vi "WPI_EncoderOpen.vi"(4 "DistancePerCount":dbl=1.0, 5 "External Reset Active High":bool=TRUE, 6 "Decoding Type":T1=enum."4x", 7 "External Reset":T2={"DevStatus"={"status"=FALSE, "code"=0, "source"=""}, "AnalogTriggerMode?"=FALSE, "DigitalMode"={"DIO Channel"=enum."Disabled"}, "AnalogTriggerMode"={"AnalogTriggerIndex"=enum."Trig 0", "OutputType"=enum."InWindow"}}, 8 "error in (no error)":errorcluster, 9 "Invert Direction (False)":bool, 10 "BSource":T2={"DevStatus"={"status"=FALSE, "code"=0, "source"=""}, "AnalogTriggerMode?"=FALSE, "DigitalMode"={"DIO Channel"=enum."Disabled"}, "AnalogTriggerMode"={"AnalogTriggerIndex"=enum."Trig 0", "OutputType"=enum."InWindow"}}, 11 "ASource":T2={"DevStatus"={"status"=FALSE, "code"=0, "source"=""}, "AnalogTriggerMode?"=FALSE, "DigitalMode"={"DIO Channel"=enum."Disabled"}, "AnalogTriggerMode"={"AnalogTriggerIndex"=enum."Trig 0", "OutputType"=enum."InWindow"}}) -> (0 "error out":errorcluster, 3 "EncoderDevRef":T6={"DevStatus"={"status"=FALSE, "code"=0, "source"=""}, "EncoderIndex"=enum."Invalid", "CounterIndex"=enum."Invalid", "DistancePerCount"=1.0, "Decoding Type"=enum."4x"})   [LabVIEW 2017]
doc: "Opens a reference to the encoder you specify. You must open a reference before using any other VIs on this palette.\n\nUse the ToDigitalSource VI to create a digital source that you can wire to the <B>ASource</B> and <B>BSource</B> inputs of this VI. After you open a reference to the encoder, you can use the Start and Stop VIs to start and stop the encoder, respectively.\n\nThis software is licensed. Open the labview\\readme\\WPI Robotics Library Open Source License.txt file for more information."
uses:
  <vilib>/Rock Robotics/SystemInterfaces/Encoder/FPGA_EncoderIdx.ctl
  <vilib>/Rock Robotics/WPI/Encoder/WPI_EncoderDevRef.ctl
  <vilib>/Rock Robotics/WPI/Encoder/WPI_EncoderCacheOp.ctl
  <vilib>/Rock Robotics/WPI/Encoder/WPI_EncoderType.ctl
  <vilib>/Rock Robotics/SystemInterfaces/Counter/FPGA_CounterCtrEdgeDetectionType.ctl
  <vilib>/Rock Robotics/SystemInterfaces/Counter/FPGA_CounterCtrSystemIndex.ctl
  <vilib>/Rock Robotics/SystemInterfaces/Encoder/FPGA_EncoderOpen & Configure.vi
  <instrlib>/Maxon Encoder/HAIOL/Simulator/Maxon Encoder Simulator.lvclass
  <vilib>/robotics/Simulator/Engine/ctl/DeviceID.ctl
  <vilib>/robotics/Simulator/NI_Robotics_Simulator.lvlib
  <vilib>/Rock Robotics/SystemInterfaces/DIO/FPGA_DIOPWMChannel.ctl
  <vilib>/Rock Robotics/SystemInterfaces/AnalogTrigger/FPGA_AnalogTriggerOutType.ctl
  <vilib>/Rock Robotics/SystemInterfaces/CounterEncoderSourceConvertion/FPGA_CounterEncoderSourceConvertionLVSourceType.ctl
  <vilib>/Rock Robotics/SystemInterfaces/DIO/FPGA_DIODigitalSourceChannel.ctl
  <vilib>/Rock Robotics/SystemInterfaces/AnalogTrigger/FPGA_AnalogTriggerIndex.ctl
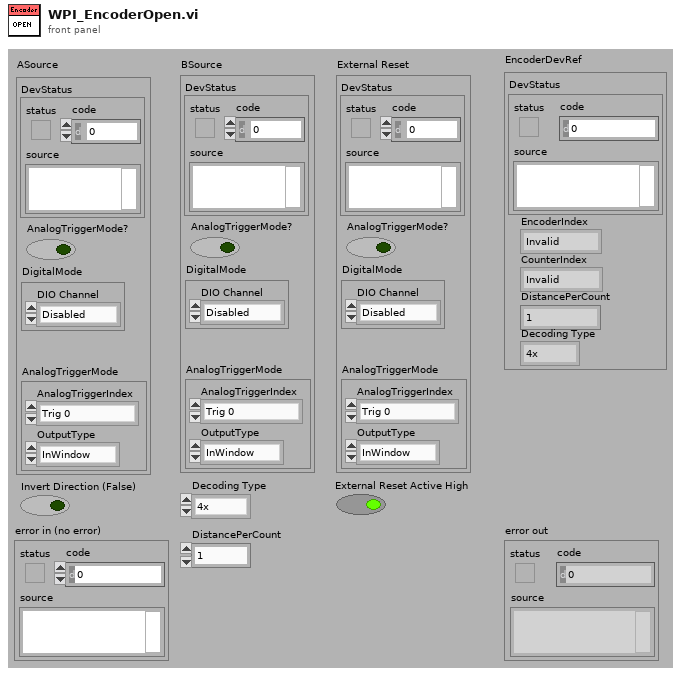
[diagram p1: front panel]
types:
  T1 = typedef "WPI_EncoderType.ctl" = enum16{"1x", "2x", "4x"}
  T2 = typedef "FPGA_CounterEncoderSourceConvertionLVSourceType.ctl" = cluster{"DevStatus":errorcluster, "AnalogTriggerMode?":bool, "DigitalMode":cluster{"DIO Channel":T3}, "AnalogTriggerMode":cluster{"AnalogTriggerIndex":T4, "OutputType":T5}}
  T3 = typedef "FPGA_DIODigitalSourceChannel.ctl" = enum8{"DIO 0", "DIO 1", "DIO 2", "DIO 3", "DIO 4", "DIO 5", "DIO 6", "DIO 7", "DIO 8", "DIO 9", "DIO MXP 0", "DIO MXP 1", "DIO MXP 2", "DIO MXP 3", "DIO MXP 4", "DIO MXP 5", "DIO MXP 6", "DIO MXP 7", "DIO MXP 8", "DIO MXP 9", "DIO MXP 10", "DIO MXP 11", "DIO MXP 12", "DIO MXP 13", "DIO MXP 14", "DIO MXP 15", "Disabled"}
  T4 = typedef "FPGA_AnalogTriggerIndex.ctl" = enum8{"Trig 0", "Trig 1", "Trig 2", "Trig 3", "Trig 4", "Trig 5", "Trig 6", "Trig 7", "Invalid"}
  T5 = typedef "FPGA_AnalogTriggerOutType.ctl" = enum16{"InWindow", "TriggerState", "Rising", "Falling"}
  T6 = typedef "WPI_EncoderDevRef.ctl" = cluster{"DevStatus":errorcluster, "EncoderIndex":T7, "CounterIndex":T8, "DistancePerCount":dbl, "Decoding Type":T1}
  T7 = typedef "FPGA_EncoderIdx.ctl" = enum8{"Enc 0", "Enc 1", "Enc 2", "Enc 3", "Enc 4", "Enc 5", "Enc 6", "Enc 7", "Invalid"}
  T8 = typedef "FPGA_CounterCtrSystemIndex.ctl" = enum8{"Ctr 0", "Ctr 1", "Ctr 2", "Ctr 3", "Ctr 4", "Ctr 5", "Ctr 6", "Ctr 7", "Invalid"}
  T9 = typedef "FPGA_CounterCtrEdgeDetectionType.ctl" = cluster{"Master Mode":enum16{"Edge Detection", "Semi Period Mode", "Pulse Length Mode", "External Direction"}, "UpChannel":enum16{"Rising Edge", "Falling Edge", "Raising & Falling Edge", "Disabled"}, "DownChannel":enum16{"Rising Edge", "Falling Edge", "Raising & Falling Edge", "Disabled"}, "High/Up":bool}
  T10 = enum16{"Rising Edge", "Falling Edge", "Raising & Falling Edge", "Disabled"}
  T11 = typedef "WPI_EncoderCacheOp.ctl" = enum16{"Acquire", "Release"}
  T12 = typedef "FPGA_DIOPWMChannel.ctl" = enum8{"PWM 0", "PWM 1", "PWM 2", "PWM 3", "PWM 4", "PWM 5", "PWM 6", "PWM 7", "PWM 8", "PWM 9", "PWM MXP 0", "PWM MXP 1", "PWM MXP 2", "PWM MXP 3", "PWM MXP 4", "PWM MXP 5", "PWM MXP 6", "PWM MXP 7", "PWM MXP 8", "PWM MXP 9", "Invalid"}
  T13 = typedef "NI_Robotics_Simulator.lvlib/DeviceID.ctl" = cluster{"robot ID":string, "sensor/actuator ID":string}
  T14 = typedef "WPI_CounterDevRef.ctl" = cluster{"DevStatus":errorcluster, "CntIndex":T8}
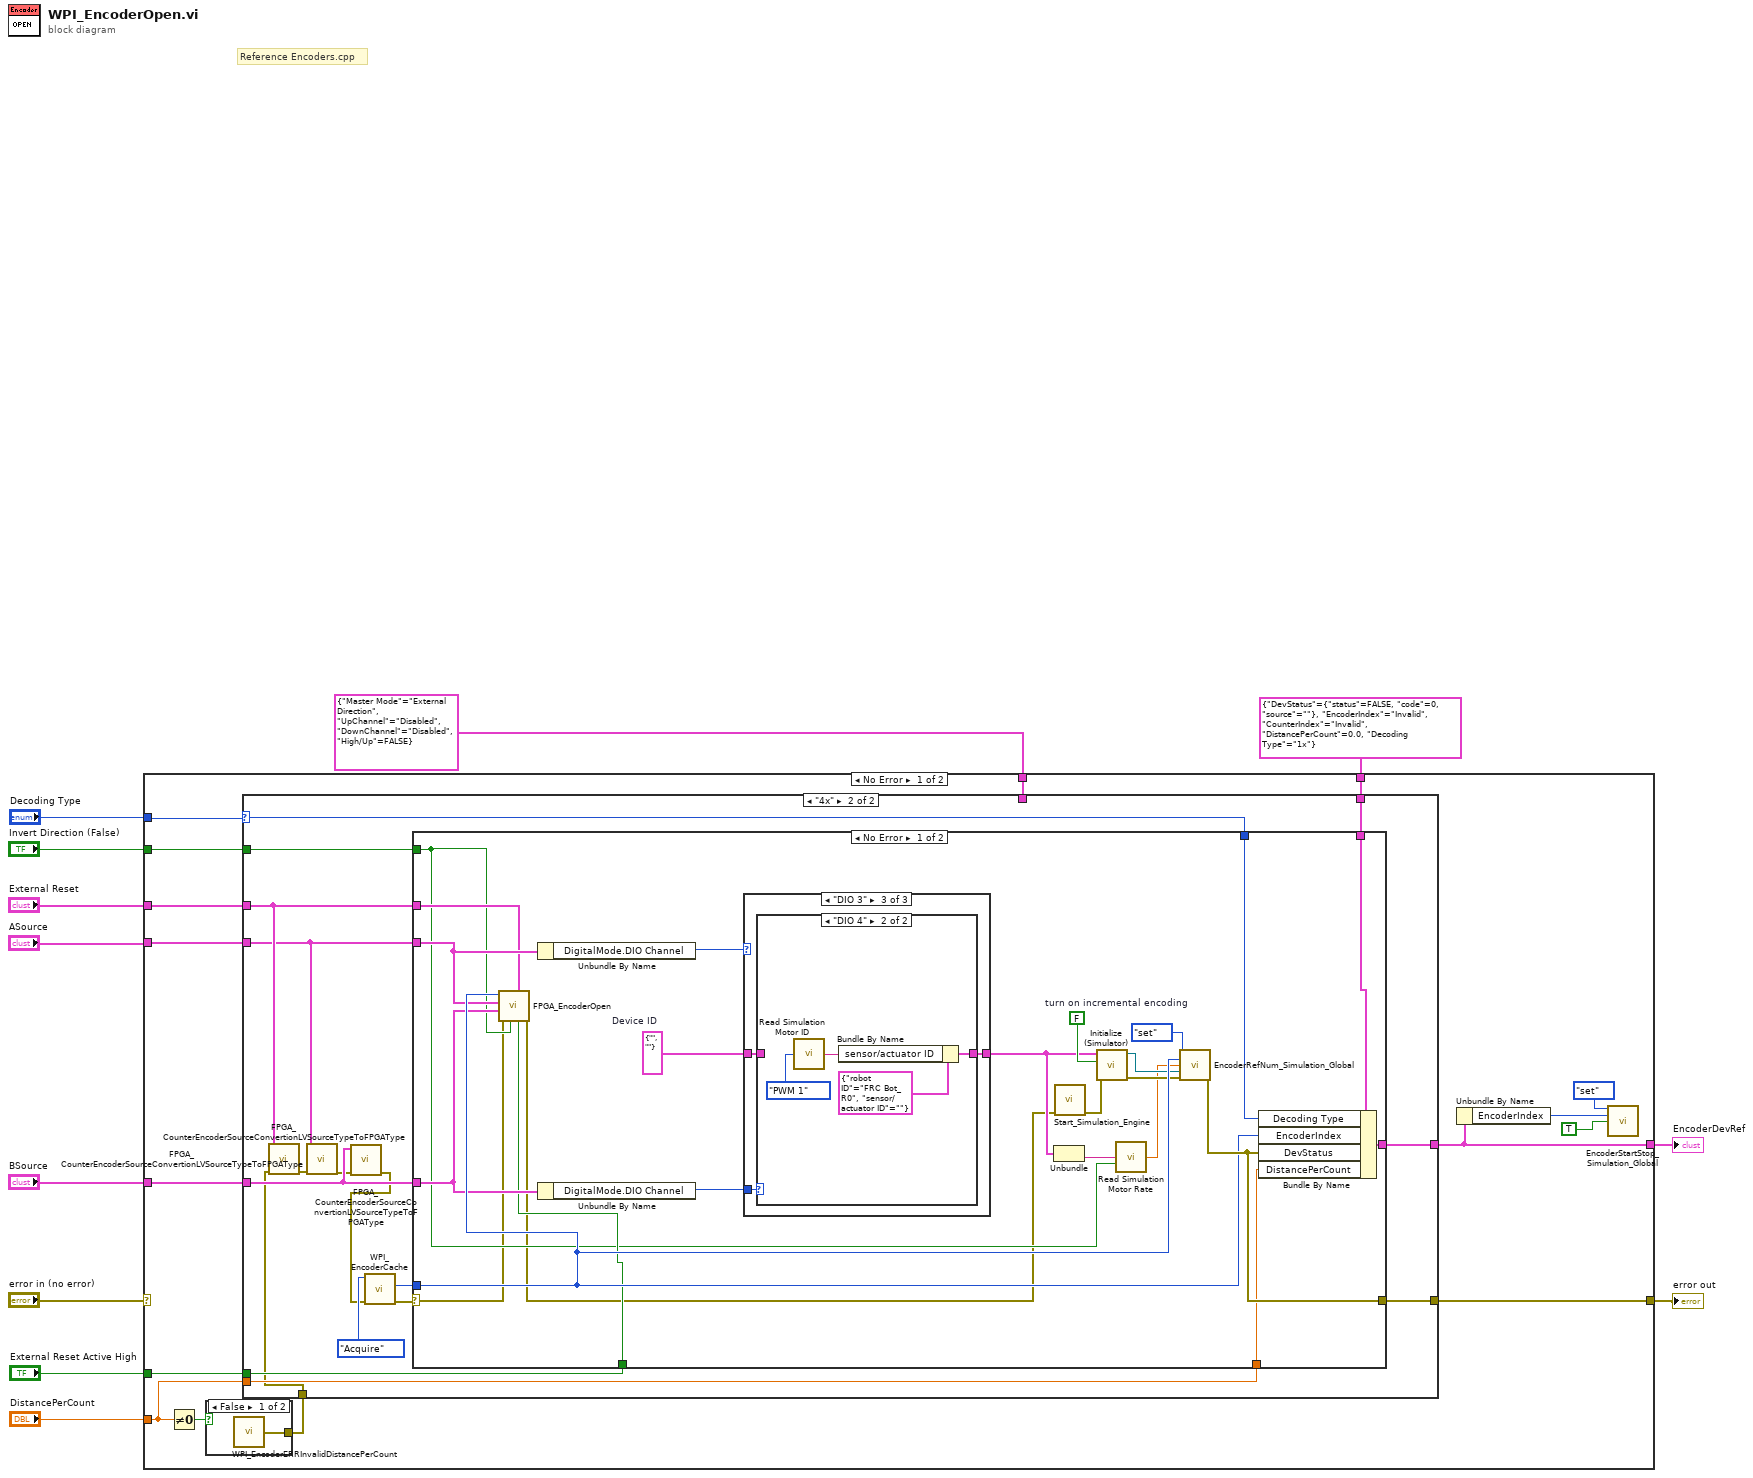
[diagram p0: block diagram]
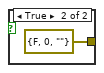
[diagram p2: hidden frame]
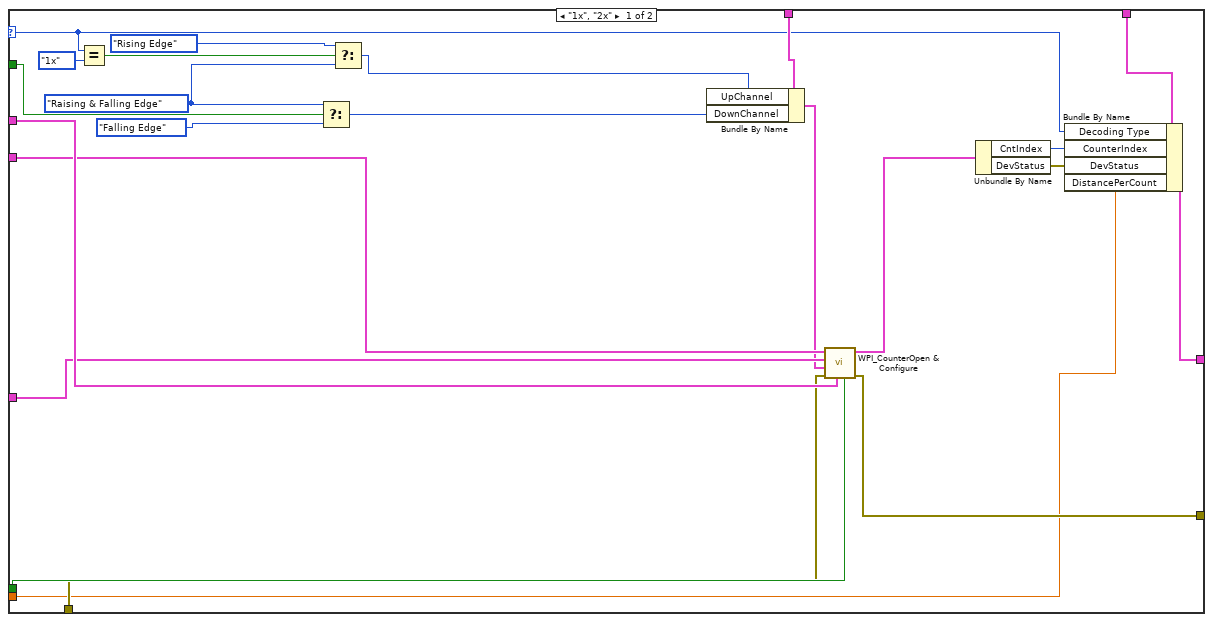
[diagram p3: hidden frame]
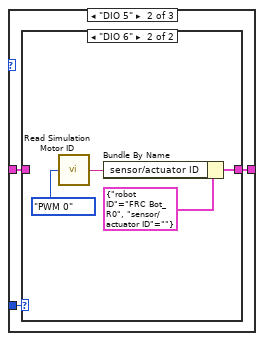
[diagram p5: hidden frame]
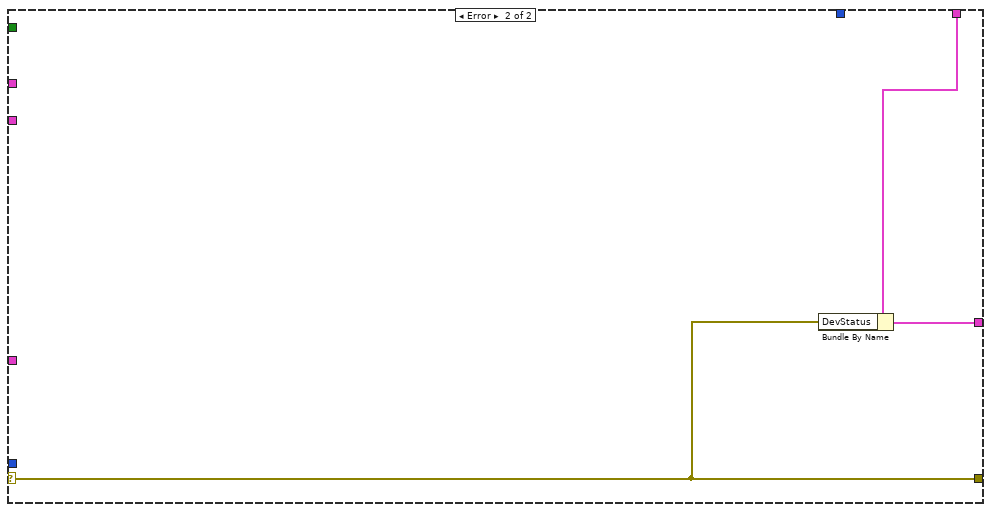
[diagram p8: hidden frame]
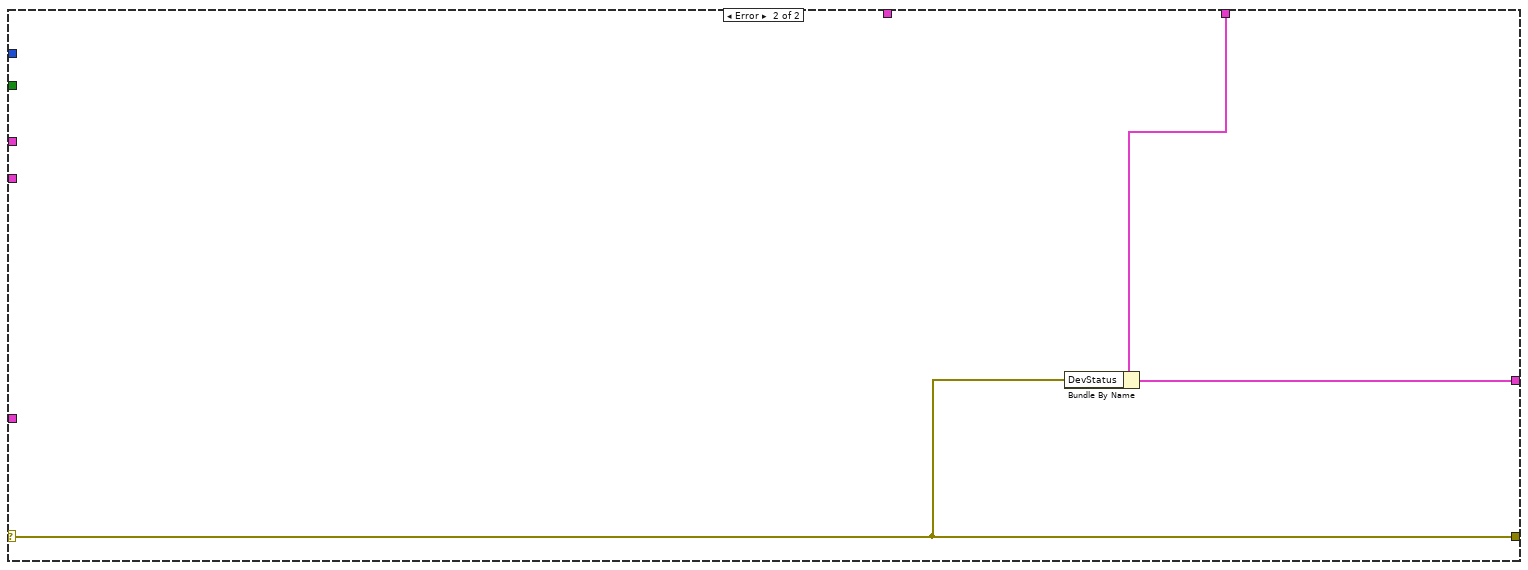
[diagram p9: hidden frame]
diagram:
  # "Reference Encoders.cpp"
  n1 = case shown="No Error" "error in (no error)" {
    selector: "error in (no error)" -> [_ w116]
    tunnel: "ASource" -> [w24 _]
    tunnel: T6 {"DevStatus"={"status"=FALSE, "code"=0, "source"=""}, "EncoderIndex"=enum."Invalid", "CounterIndex"=enum."Invalid", "DistancePerCount"=0.0, "Decoding Type"=enum."1x"} ("QuadEncoderDevRef") -> [w28 w117]
    tunnel: [w16 w115] -> w10
    tunnel: [w27 w116] -> w9
    tunnel: "Invert Direction (False)" -> [w26 _]
    tunnel: "BSource" -> [w25 _]
    tunnel: "External Reset" -> [w19 _]
    tunnel: "External Reset Active High" -> [w23 _]
    tunnel: "Decoding Type" -> [w22 _]
    tunnel: "DistancePerCount" -> [w21 _]
    tunnel: T9 {"Master Mode"=enum."External Direction", "UpChannel"=enum."Disabled", "DownChannel"=enum."Disabled", "High/Up"=FALSE} ("EdgeType") -> [w20 _]
    frame No Error {
      n2 = Not Equal To 0?(x=w21) -> (x != 0?=w18:bool)
      n3 = case shown="False" w18 {
        tunnel: [w29 errorcluster {"status"=FALSE, "code"=0, "source"=""} ("f")] -> w17
        frame False {
          n4 = call <vilib>:"WPI_EncoderERRInvalidDistancePerCount.vi"() -> ("ERRInvalidDistancePerCount"=w29:errorcluster)
        }
        frame True {
        }
      }
      n5 = case shown="\"4x\"" w22 {
        selector: w22 -> [w42 w62]
        tunnel: w28 -> [w44 w67]
        tunnel: [w34 w66] -> w16
        tunnel: [w49 w65] -> w27
        tunnel: w26 -> [w41 w64]
        tunnel: w25 -> [w51 w59]
        tunnel: w24 -> [w52 w58]
        tunnel: w19 -> [w53 w60]
        tunnel: w23 -> [w50 w63]
        tunnel: w21 -> [w33 w61]
        tunnel: w20 -> [w48 _]
        tunnel: w17 -> [w43 w54]
        frame "1x", "2x" {
          w31 = T10."Raising & Falling Edge" ("DownChannel")
          n6 = Equal?(x=w42, y=WPI_EncoderType."1x" ("Decoding Type")) -> (x = y?=w40:bool)
          n7 = Select(t=w31, s=w41, f=T10."Falling Edge" ("DownChannel")) -> (s? t:f=w45:T10)
          n8 = Select(t=T10."Rising Edge", s=w40, f=w31) -> (s? t:f=w39:T10)
          n9 = Bundle By Name(cluster=w48, "UpChannel"=w39, "DownChannel"=w45) -> (w47:T9)
          n10 = call <vilib>:"WPI_CounterOpen & Configure.vi"("External Reset Trigger"=w50, "External Reset"=w53, "error in (no error)"=w43, "EdgeType"=w47, "Down Source"=w51, "Up Source"=w52) -> ("error out"=w49:errorcluster, "CounterDevRef"=w37:T14)  [unwired: 4 out]
          n11 = Unbundle By Name(w37) -> ("CntIndex"=w36:T8, "DevStatus"=w35:errorcluster)
          n12 = Bundle By Name(cluster=w44, "Decoding Type"=w42, "CounterIndex"=w36, "DevStatus"=w35, "DistancePerCount"=w33) -> (w34:T6)
        }
        frame "4x" {
          n13 = call <vilib>:"FPGA_CounterEncoderSourceConvertionLVSourceTypeToFPGAType.vi"("error in (no error)"=w54, "DigitalSource"=w60) -> ("error out"=w57:errorcluster)  [unwired: 9 out]
          n14 = call <vilib>:"FPGA_CounterEncoderSourceConvertionLVSourceTypeToFPGAType.vi"("error in (no error)"=w57, "DigitalSource"=w58) -> ("error out"=w56:errorcluster)  [unwired: 9 out]
          n15 = call <vilib>:"FPGA_CounterEncoderSourceConvertionLVSourceTypeToFPGAType.vi"("error in (no error)"=w56, "DigitalSource"=w59) -> ("error out"=w55:errorcluster)  [unwired: 9 out]
          n16 = call <vilib>:"WPI_EncoderCache.vi"("error in (no error)"=w55, "Operation"=WPI_EncoderCacheOp."Acquire") -> ("error out"=w69:errorcluster, "EncoderAllocated"=w68:T7)  [unwired: 1 in, 7 out]
          n17 = case shown="No Error" w69 {
            selector: w69 -> [w72 w114]
            tunnel: [w94 w112] -> w66
            tunnel: [w92 w114] -> w65
            tunnel: w67 -> [w93 w113]
            tunnel: w68 -> [w91 _]
            tunnel: w64 -> [w84 _]
            tunnel: w58 -> [w90 _]
            tunnel: w59 -> [w89 _]
            tunnel: w60 -> [w88 _]
            tunnel: w63 -> [w87 _]
            tunnel: w61 -> [w86 _]
            tunnel: w62 -> [w85 _]
            frame No Error {
              w76 = FALSE  # turn on incremental encoding
              w83 = T13 {"robot ID"="", "sensor/actuator ID"=""}  # Device ID
              n18 = call-poly <vilib>:"FPGA_EncoderOpen.vi"("IndexActiveHigh"=w87, "IndexSource"=w88, "Reverse?"=w84, "error in"=w72, "BSource"=w89, "ASource"=w90, "EncoderIndex"=w91) -> ("error out"=w71:errorcluster)  [unwired: 1 in, 3 out]
              n19 = Unbundle By Name(w90) -> ("DigitalMode.DIO Channel"=w77:T3)
              n20 = Unbundle By Name(w89) -> ("DigitalMode.DIO Channel"=w79:T3)
              n21 = case shown="\"DIO 3\"" w77 {
                tunnel: w83 -> [w95 w97 w105]
                tunnel: w79 -> [_ w98 w106]
                tunnel: [w95 w96 w104] -> w75
                frame Default {
                }
                frame "DIO 5" {
                  n22 = case shown="\"DIO 6\"" w98 {
                    tunnel: w97 -> [w99 _]
                    tunnel: [w99 w101] -> w96
                    frame Default {
                    }
                    frame "DIO 6" {
                      n23 = call <vilib>:"Read Simulation Motor ID.vi"("PWM.PWM Channel"=FPGA_DIOPWMChannel."PWM 0") -> ("motor ID"=w103:string)  [unwired: 13 in, 1 out]
                      n24 = Bundle By Name(cluster=T13 {"robot ID"="FRC Bot_R0", "sensor/actuator ID"=""} ("Device ID"), "sensor/actuator ID"=w103) -> (w101:T13)
                    }
                  }
                }
                frame "DIO 3" {
                  n25 = case shown="\"DIO 4\"" w106 {
                    tunnel: w105 -> [w107 _]
                    tunnel: [w107 w109] -> w104
                    frame Default {
                    }
                    frame "DIO 4" {
                      n26 = call <vilib>:"Read Simulation Motor ID.vi"("PWM.PWM Channel"=FPGA_DIOPWMChannel."PWM 1") -> ("motor ID"=w111:string)  [unwired: 13 in, 1 out]
                      n27 = Bundle By Name(cluster=T13 {"robot ID"="FRC Bot_R0", "sensor/actuator ID"=""} ("Device ID"), "sensor/actuator ID"=w111) -> (w109:T13)
                    }
                  }
                }
              }
              n28 = Unbundle(w75) -> ("sensor/actuator ID"=w73:string)  [unwired: 1 out]
              n29 = call <vilib>:"Start_Simulation_Engine.vi"("error in"=w71) -> ("error out"=w82:errorcluster)  [unwired: 14 in]
              n30 = call <instrlib>:"Initialize (Simulator).vi"("error in (no error)"=w82, "Z Index Enabled (F:Disable)"=w76, "Device ID"=w75) -> ("error out"=w81:errorcluster, "Maxon Encoder out"=w80:refnum<class "Maxon Encoder.lvclass">)  [unwired: 7 in]
              n31 = call <vilib>:"Read Simulation Motor Rate.vi"("motor ID"=w73, "Invert Direction (False)"=w84) -> ("Rate"=w74:dbl)  [unwired: 12 in, 1 out]
              n32 = call <vilib>:"EncoderRefNum_Simulation_Global.vi"("menu"=enum16{"set", "get", "delete"}."set", "Encoder"=w91, "Rate in"=w74, "Maxon Encoder Set"=w80, "error in (no error)"=w81) -> ("error out"=w92:errorcluster)  [unwired: 8 in, 2 out]
              n33 = Bundle By Name(cluster=w93, "Decoding Type"=w85, "EncoderIndex"=w91, "DevStatus"=w92, "DistancePerCount"=w86) -> (w94:T6)
            }
            frame Error {
              n34 = Bundle By Name(cluster=w113, "DevStatus"=w114) -> (w112:T6)
            }
          }
        }
      }
      n35 = Unbundle By Name(w16) -> ("EncoderIndex"=w13:T7)
      n36 = call <vilib>:"EncoderStartStop_Simulation_Global.vi"("menu"=enum16{"set", "get", "delete"}."set", "Encoder Index"=w13, "start/stop in"=TRUE ("Enable")) -> ()  [unwired: 11 in, 2 out]
    }
    frame Error {
      n37 = Bundle By Name(cluster=w117, "DevStatus"=w116) -> (w115:T6)
    }
  }
  "EncoderDevRef" <- w10
  "error out" <- w9
